vi "SawtoothSubVi.vi"(6 "Error In":errorcluster, 8 "Frequency":dbl, 9 "DC Offset":dbl, 10 "Duty Cycle":dbl, 11 "Amp":dbl) -> (0 "Error Out":errorcluster, 3 "Array":dbl[](array[numeric]))   [LabVIEW 2017]
panel:
  out "Waveform Graph":dbl[](graph)
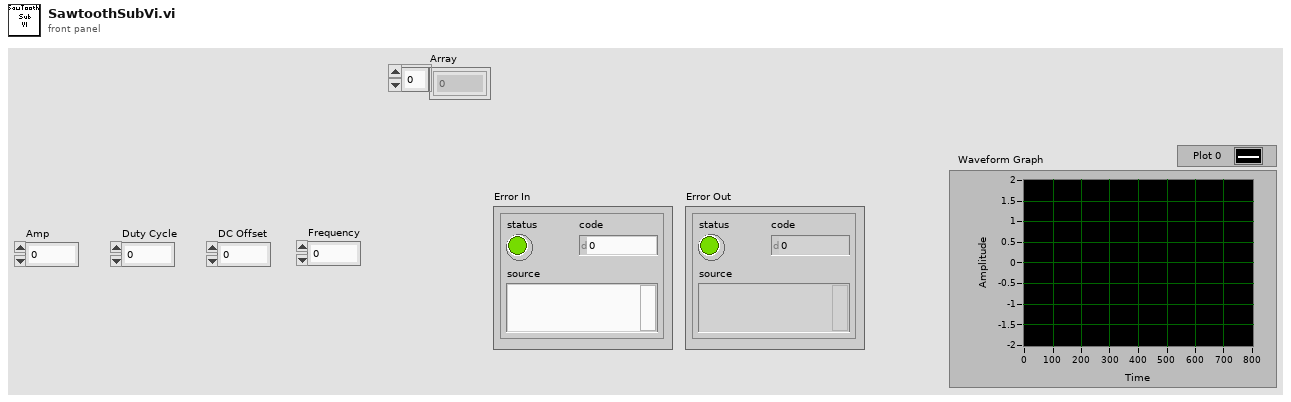
[diagram p1: front panel]
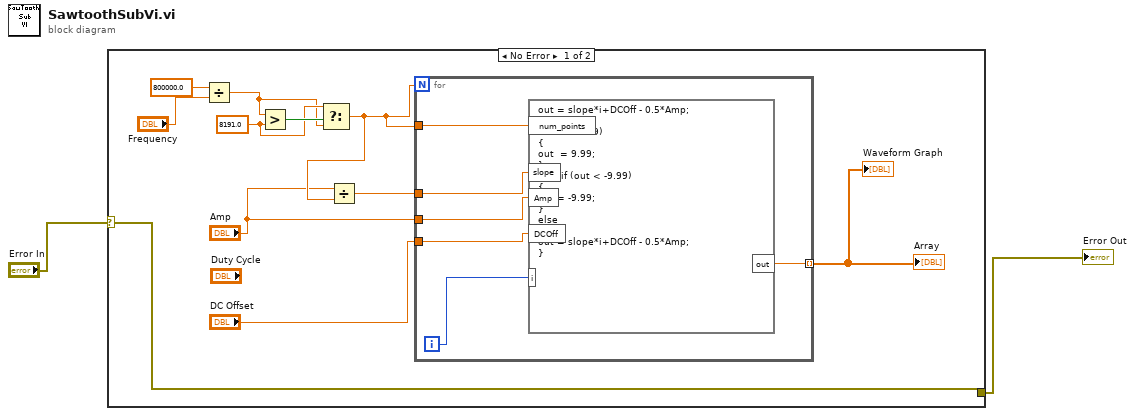
[diagram p0: block diagram]
diagram:
  n1 = case shown="No Error" "Error In" {
    selector: "Error In" -> [w13 w20]
    tunnel: [w13 w20] -> w1
    frame No Error {
      w9 = 8191.0 ("y")
      n2 = Divide(x=800000.0, y="Frequency") -> (x/y=w8:dbl)
      n3 = Greater?(x=w8, y=w9) -> (0:w10:bool)
      n4 = Select(t=w9, s=w10, f=w8) -> (s? t:f=w6:dbl)
      n5 = Divide(x="Amp", y=w6) -> (x/y=w7:dbl)
      n6 = for {
        N: w6 -> [_]
        tunnel: w6 -> [w19]
        tunnel: w7 -> [w18]
        tunnel: [w17] -> w3 mode=indexing
        tunnel: "DC Offset" -> [w15]
        tunnel: "Amp" -> [w14]
        i -> [w16]
        n7 = formula code="out = slope*i+DCOff - 0.5*Amp;\n\nif(out > 9.99)\n{\nout  = 9.99;\n}\nelse if (out < -9.99)\n{\nout = -9.99;\n}\nelse\n{\nout = slope*i+DCOff - 0.5*Amp;\n}"("num_points"=w19, "slope"=w18, "i"=w16, "DCOff"=w15, "Amp"=w14) -> ("out"=w17:dbl)
      }
      "Array" <- w3
      "Waveform Graph" <- w3
    }
    frame Error {
    }
  }
  "Error Out" <- w1
